vi "SweepOver.vi"(0 "VISA resource name":refnum<visa-resource-name>="LIA", 1 "Sweep Over":string(combo)="Internal Freq", 2 "Sweep Mode":string(combo)="Logarithmic", 3 "End Mode":string(combo)="0", 5 "error in (no error)":errorcluster, 6 "SubVI":bool, 7 "Sweep Time":dbl=100.0 min=0.0 format="%#.4g", 8 "?":bool, 9 "Update Interval":string(combo)="0", 10 "Single Lock-in Parameter 1 (0: X output)":i32(ring)=15 items=["X output", "Y output", "R output", "Theta output", "Aux In 1", "Aux In 2", "Aux In 3", "Aux In 4", "Aux Out 1", "Aux Out 2", "Xnoise", "Ynoise", "Reference Phase", "Sine Out Amplitude", "DC Level", "Int. Ref. Frequency", "Ext. Ref. Frequency"], 11 "Sweep Start":dbl=0.001 min=0.001 max=2500000.0, 12 "Single Lock-in Parameter 2 (0: X output)":i32(ring)=2 items=["X output", "Y output", "R output", "Theta output", "Aux In 1", "Aux In 2", "Aux In 3", "Aux In 4", "Aux Out 1", "Aux Out 2", "Xnoise", "Ynoise", "Reference Phase", "Sine Out Amplitude", "DC Level", "Int. Ref. Frequency", "Ext. Ref. Frequency"], 13 "Sweep End":dbl=2500000.0 min=0.001 max=2500000.0) -> (14 "VISA resource name out":refnum<visa-resource-name>, 15 "output cluster":cluster{dbl[], dbl[]}, 19 "error out":errorcluster)   [LabVIEW 2016]
uses:
  <instrlib>/Stanford Research SR865/Stanford Research SR865.lvlib
panel:
  out "Scan State 2":i32(ring) items=["Off or Disabled", "Reset", "Running", "Paused", "Done"]
  out "?":string="Hz"
  out "?":string="Hz"
  # "s"
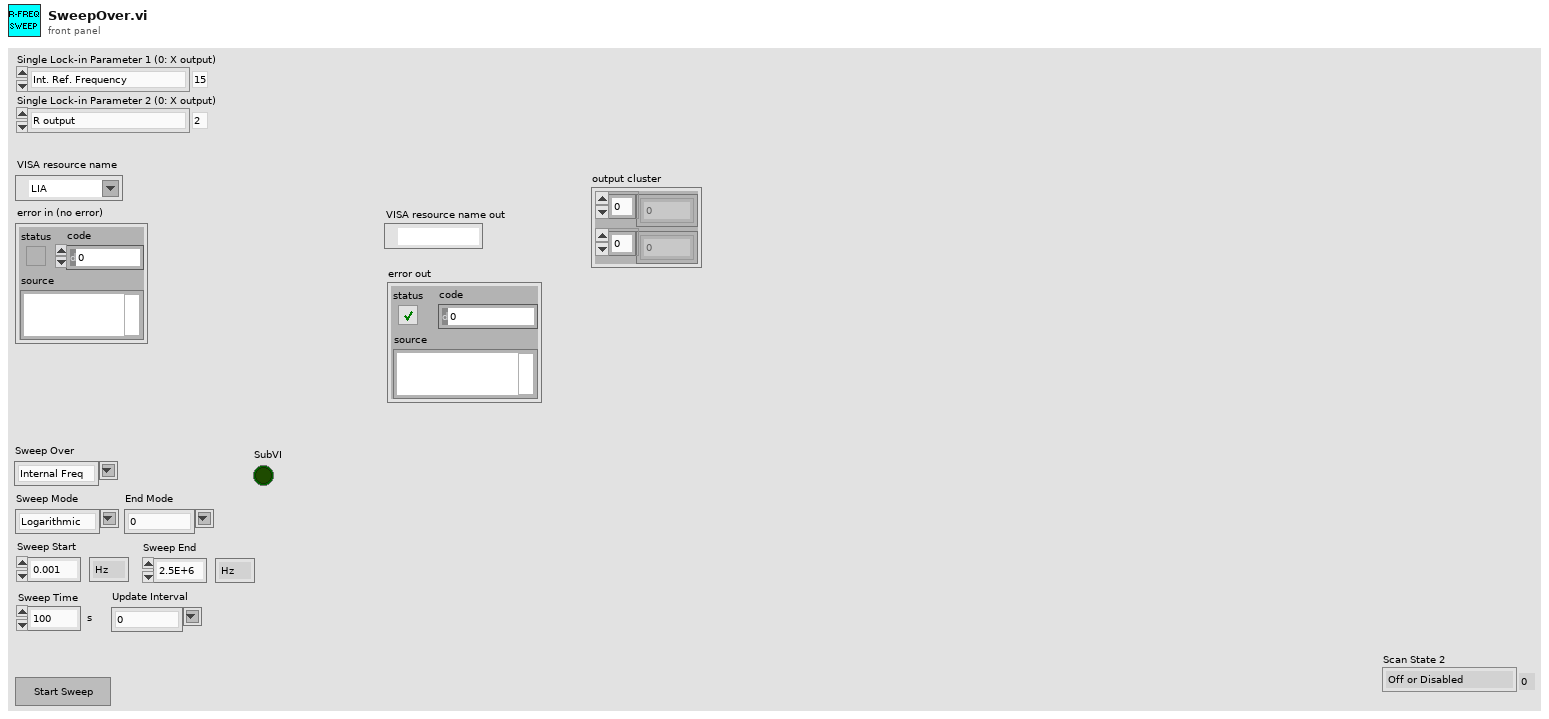
[diagram p1: front panel]
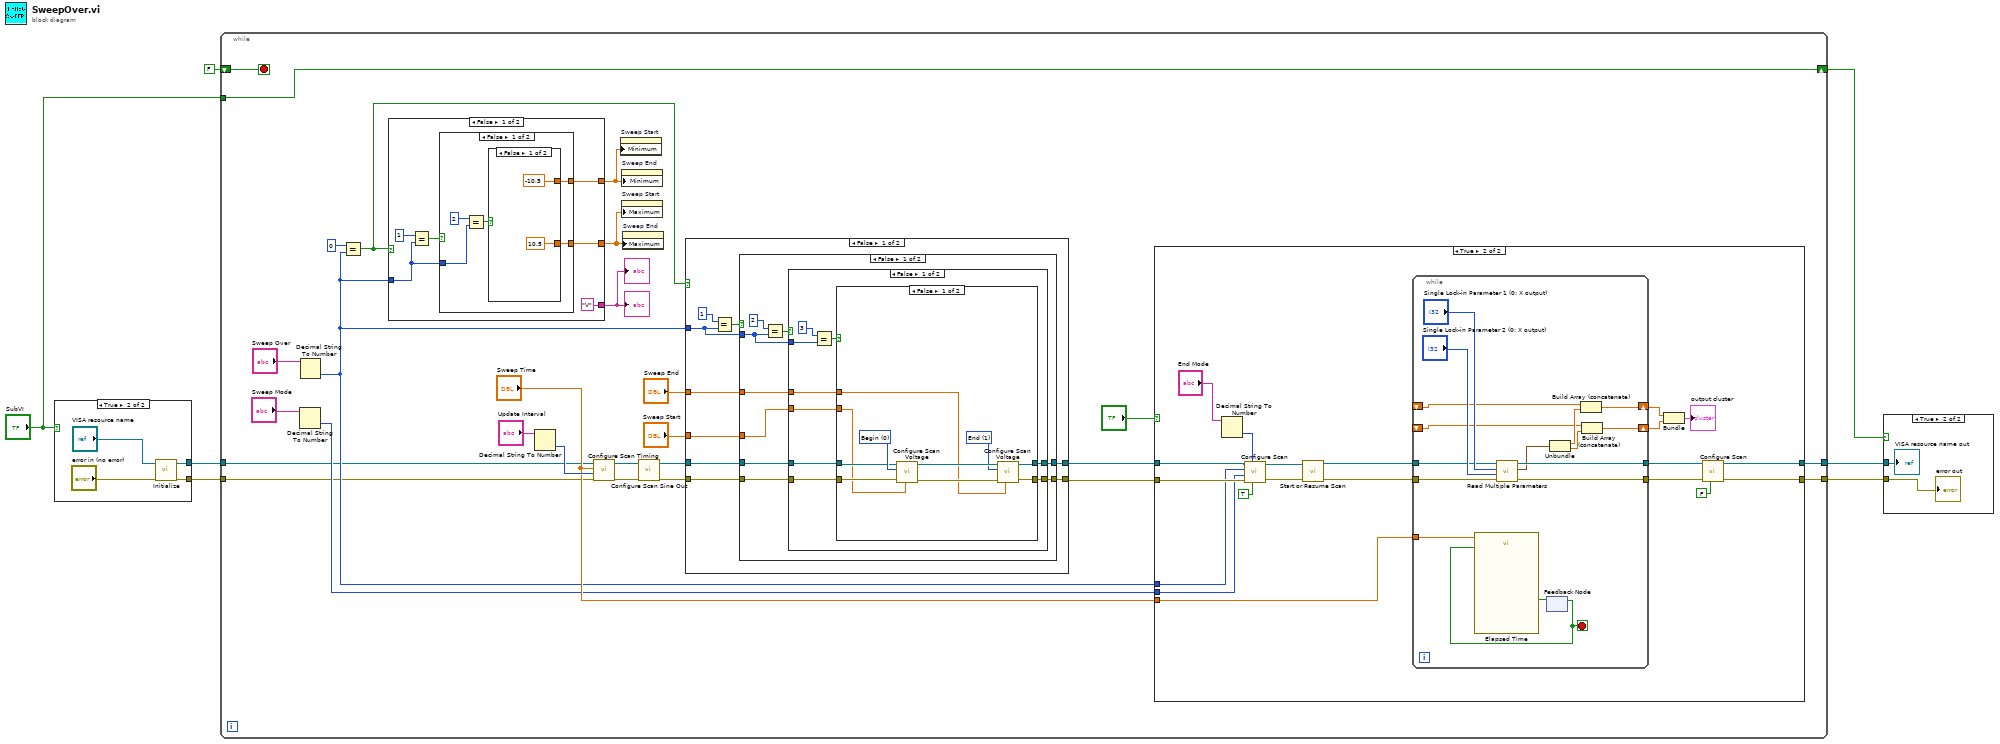
[diagram p0: block diagram]
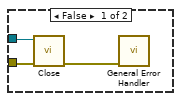
[diagram p2: hidden frame]
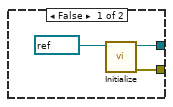
[diagram p3: hidden frame]
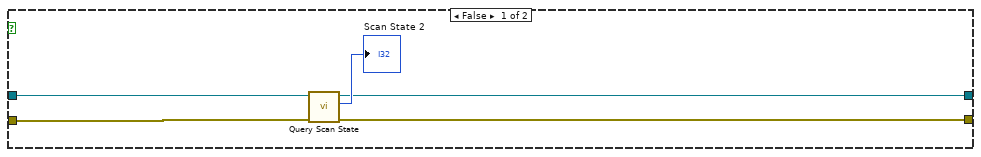
[diagram p4: hidden frame]
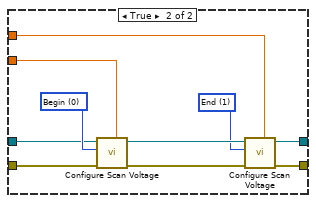
[diagram p5: hidden frame]
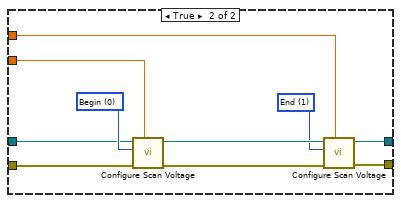
[diagram p6: hidden frame]
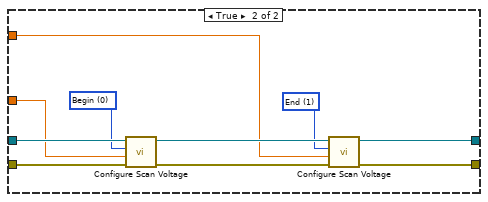
[diagram p7: hidden frame]
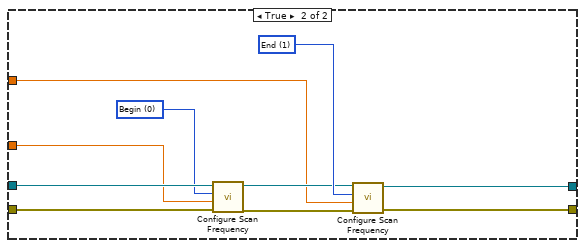
[diagram p8: hidden frame]
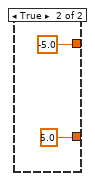
[diagram p9: hidden frame]
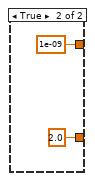
[diagram p10: hidden frame]
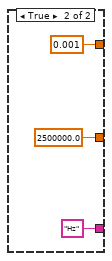
[diagram p11: hidden frame]
diagram:
  n1 = case shown="True" "SubVI" {
    tunnel: [w9 w14] -> w7
    tunnel: [w8 w13] -> w6
    frame False {
      n2 = call <instrlib>:"Initialize.vi"("VISA resource name"=refnum<visa-resource-name> "LIA") -> ("error out"=w8:errorcluster, "VISA resource name out"=w9:refnum<visa-resource-name>)  [unwired: 9 in]
    }
    frame True {
      n3 = call <instrlib>:"Initialize.vi"("error in (no error)"="error in (no error)", "VISA resource name"="VISA resource name") -> ("error out"=w13:errorcluster, "VISA resource name out"=w14:refnum<visa-resource-name>)  [unwired: 8 in]
    }
  }
  n4 = while {
    tunnel: w7 -> [w18]
    tunnel: w6 -> [w17]
    tunnel: [w25] -> w3
    tunnel: [w24] -> w4
    shift-right: [w15] -> w1
    shift-left: FALSE ("SubVI") -> [w23]
    tunnel: "SubVI" -> [w15]
    stop <- w23 stop-if-true
    n5 = Decimal String To Number(string="Sweep Mode") -> (number=w19:i32)  [unwired: 2 in, 1 out]
    n6 = Decimal String To Number(string="Sweep Over") -> (number=w20:i32)  [unwired: 2 in, 1 out]
    n7 = Equal?(x=0, y=w20) -> (x = y?=w29:bool)
    n8 = case shown="False" w29 {
      tunnel: ["V" "Hz"] -> w32
      tunnel: w20 -> [w160 _]
      tunnel: [w162 0.001 ("Data Entry Limits:Minimum")] -> w28
      tunnel: [w161 2500000.0 ("Data Entry Limits:Maximum")] -> w27
      frame False {
        n9 = Equal?(x=1, y=w160) -> (x = y?=w163:bool)
        n10 = case shown="False" w163 {
          tunnel: [w170 1e-09 ("Data Entry Limits:Maximum")] -> w162
          tunnel: [w169 2.0 ("Data Entry Limits:Minimum")] -> w161
          tunnel: w160 -> [w167 _]
          frame False {
            n11 = Equal?(x=2, y=w167) -> (x = y?=w166:bool)
            n12 = case shown="False" w166 {
              tunnel: [-10.5 ("Data Entry Limits:Maximum") -5.0 ("Data Entry Limits:Maximum")] -> w170
              tunnel: [10.5 ("Data Entry Limits:Minimum") 5.0 ("Data Entry Limits:Minimum")] -> w169
              frame False {
              }
              frame True {
              }
            }
          }
          frame True {
          }
        }
      }
      frame True {
      }
    }
    "?" <- w32
    "?" <- w32
    n13 = Decimal String To Number(string="Update Interval") -> (number=w35:i32)  [unwired: 2 in, 1 out]
    n14 = call <instrlib>:"Configure Scan Timing.vi"("error in (no error)"=w17, "Update Interval (0: 8ms)"=w35, "Scan Time (100)"="Sweep Time", "VISA resource name"=w18) -> ("error out"=w40:errorcluster, "VISA resource name out"=w41:refnum<visa-resource-name>)  [unwired: 6 in]
    n15 = property on="Sweep Start" class="DigNum (strict)"("Minimum"=w28) -> ()  [unwired: 2 in, 2 out]
    n16 = property on="Sweep End" class="DigNum (strict)"("Minimum"=w28) -> ()  [unwired: 2 in, 2 out]
    n17 = property on="Sweep Start" class="DigNum (strict)"("Maximum"=w27) -> ()  [unwired: 2 in, 2 out]
    n18 = property on="Sweep End" class="DigNum (strict)"("Maximum"=w27) -> ()  [unwired: 2 in, 2 out]
    n19 = call <instrlib>:"Configure Scan Sine Out.vi"("error in (no error)"=w40, "VISA resource name"=w41) -> ("error out"=w38:errorcluster, "VISA resource name out"=w39:refnum<visa-resource-name>)  [unwired: 8 in]
    n20 = case shown="False" w29 {
      tunnel: w39 -> [w91 w159]
      tunnel: w38 -> [w90 w158]
      tunnel: [w89 w153] -> w22
      tunnel: [w88 w152] -> w21
      tunnel: "Sweep Start" -> [w84 w151]
      tunnel: "Sweep End" -> [w85 w150]
      tunnel: w20 -> [w83 _]
      frame False {
        n21 = Equal?(x=1, y=w83) -> (x = y?=w86:bool)
        n22 = case shown="False" w86 {
          tunnel: w91 -> [w100 w149]
          tunnel: w90 -> [w99 w148]
          tunnel: [w98 w145] -> w89
          tunnel: [w97 w144] -> w88
          tunnel: w85 -> [w93 w140]
          tunnel: w84 -> [w94 w141]
          tunnel: w83 -> [w92 _]
          frame False {
            n23 = Equal?(x=2, y=w92) -> (x = y?=w95:bool)
            n24 = case shown="False" w95 {
              tunnel: w100 -> [w103 w135]
              tunnel: w99 -> [w104 w134]
              tunnel: [w106 w133] -> w98
              tunnel: [w105 w132] -> w97
              tunnel: w94 -> [w102 w131]
              tunnel: w93 -> [w101 w130]
              tunnel: w92 -> [w108 _]
              frame False {
                n25 = Equal?(x=3, y=w108) -> (x = y?=w107:bool)
                n26 = case shown="False" w107 {
                  tunnel: [w114 w125] -> w106
                  tunnel: [w115 w124] -> w105
                  tunnel: w104 -> [w112 w123]
                  tunnel: w103 -> [w113 w122]
                  tunnel: w102 -> [w111 w121]
                  tunnel: w101 -> [w110 w120]
                  frame False {
                    w116 = 1 items=["Begin", "End"] ("Scan Begin or End (0: Begin)")
                    w117 = 0 items=["Begin", "End"] ("Scan Begin or End (0: Begin)")
                    n27 = call <instrlib>:"Configure Scan Voltage.vi"("AuxOut2 to Voltage (2)"=w111, "error in (no error)"=w112, "Scan Begin or End (0: Begin)"=w117, "VISA resource name"=w113) -> ("error out"=w119:errorcluster, "VISA resource name out"=w118:refnum<visa-resource-name>)  [unwired: 6 in]
                    n28 = call <instrlib>:"Configure Scan Voltage.vi"("AuxOut2 to Voltage (2)"=w110, "error in (no error)"=w119, "Scan Begin or End (0: Begin)"=w116, "VISA resource name"=w118) -> ("error out"=w115:errorcluster, "VISA resource name out"=w114:refnum<visa-resource-name>)  [unwired: 6 in]
                  }
                  frame True {
                    w126 = 1 items=["Begin", "End"] ("Scan Begin or End (0: Begin)")
                    w127 = 0 items=["Begin", "End"] ("Scan Begin or End (0: Begin)")
                    n29 = call <instrlib>:"Configure Scan Voltage.vi"("AuxOut 1 to Voltage (-2)"=w121, "error in (no error)"=w123, "Scan Begin or End (0: Begin)"=w127, "VISA resource name"=w122) -> ("error out"=w129:errorcluster, "VISA resource name out"=w128:refnum<visa-resource-name>)  [unwired: 6 in]
                    n30 = call <instrlib>:"Configure Scan Voltage.vi"("AuxOut 1 to Voltage (-2)"=w120, "error in (no error)"=w129, "Scan Begin or End (0: Begin)"=w126, "VISA resource name"=w128) -> ("error out"=w124:errorcluster, "VISA resource name out"=w125:refnum<visa-resource-name>)  [unwired: 6 in]
                  }
                }
              }
              frame True {
                w136 = 1 items=["Begin", "End"] ("Scan Begin or End (0: Begin)")
                w137 = 0 items=["Begin", "End"] ("Scan Begin or End (0: Begin)")
                n31 = call <instrlib>:"Configure Scan Voltage.vi"("DC Level to Voltage (-1)"=w131, "error in (no error)"=w134, "Scan Begin or End (0: Begin)"=w137, "VISA resource name"=w135) -> ("error out"=w139:errorcluster, "VISA resource name out"=w138:refnum<visa-resource-name>)  [unwired: 6 in]
                n32 = call <instrlib>:"Configure Scan Voltage.vi"("DC Level to Voltage (-1)"=w130, "error in (no error)"=w139, "Scan Begin or End (0: Begin)"=w136, "VISA resource name"=w138) -> ("error out"=w132:errorcluster, "VISA resource name out"=w133:refnum<visa-resource-name>)  [unwired: 6 in]
              }
            }
          }
          frame True {
            w142 = 1 items=["Begin", "End"] ("Scan Begin or End (0: Begin)")
            w143 = 0 items=["Begin", "End"] ("Scan Begin or End (0: Begin)")
            n33 = call <instrlib>:"Configure Scan Voltage.vi"("error in (no error)"=w148, "Amplitude to Voltage (1)"=w141, "Scan Begin or End (0: Begin)"=w143, "VISA resource name"=w149) -> ("error out"=w147:errorcluster, "VISA resource name out"=w146:refnum<visa-resource-name>)  [unwired: 6 in]
            n34 = call <instrlib>:"Configure Scan Voltage.vi"("error in (no error)"=w147, "Amplitude to Voltage (1)"=w140, "Scan Begin or End (0: Begin)"=w142, "VISA resource name"=w146) -> ("error out"=w144:errorcluster, "VISA resource name out"=w145:refnum<visa-resource-name>)  [unwired: 6 in]
          }
        }
      }
      frame True {
        w156 = 1 items=["Begin", "End"] ("Scan Begin or End (0: Begin)")
        w157 = 0 items=["Begin", "End"] ("Scan Begin or End (0: Begin)")
        n35 = call <instrlib>:"Configure Scan Frequency.vi"("error in (no error)"=w158, "Frequency (100000)"=w151, "Scan Begin or End (0: Begin)"=w157, "VISA resource name"=w159) -> ("error out"=w154:errorcluster, "VISA resource name out"=w155:refnum<visa-resource-name>)  [unwired: 6 in]
        n36 = call <instrlib>:"Configure Scan Frequency.vi"("error in (no error)"=w154, "Frequency (100000)"=w150, "Scan Begin or End (0: Begin)"=w156, "VISA resource name"=w155) -> ("error out"=w152:errorcluster, "VISA resource name out"=w153:refnum<visa-resource-name>)  [unwired: 6 in]
      }
    }
    n37 = case shown="True" "?" {
      tunnel: "Sweep Time" -> [_ w65]
      tunnel: [w42 w52] -> w25
      tunnel: [w43 w51] -> w24
      tunnel: w22 -> [w45 w62]
      tunnel: w21 -> [w44 w61]
      tunnel: w20 -> [_ w60]
      tunnel: w19 -> [_ w59]
      frame False {
        n38 = call <instrlib>:"Query Scan State.vi"("error in (no error)"=w44, "VISA resource name"=w45) -> ("error out"=w43:errorcluster, "Scan State"=→"Scan State 2":i32, "VISA resource name out"=w42:refnum<visa-resource-name>)  [unwired: 7 in]
      }
      frame True {
        n39 = Decimal String To Number(string="End Mode") -> (number=w58:i32)  [unwired: 2 in, 1 out]
        n40 = call <instrlib>:"Configure Scan.vi"("Scanning State (0: Off)"=TRUE, "Scan End Mode (0: Once)"=w58, "error in (no error)"=w61, "Scan Type (0: Linear)"=w59, "Scan Parameter (0: Fint)"=w60, "VISA resource name"=w62) -> ("error out"=w64:errorcluster, "VISA resource name out"=w63:refnum<visa-resource-name>)  [unwired: 4 in]
        n41 = call <instrlib>:"Start or Resume Scan.vi"("error in (no error)"=w64, "VISA resource name"=w63) -> ("error out"=w47:errorcluster, "VISA resource name out"=w48:refnum<visa-resource-name>)  [unwired: 8 in]
        n42 = while {
          tunnel: w65 -> [w80]
          tunnel: [w78] -> w50
          tunnel: [w79] -> w49
          shift-right: [w72] -> w56
          shift-left: _ -> [w69]
          shift-right: [w71] -> w55
          shift-left: _ -> [w70]
          tunnel: w48 -> [w68]
          tunnel: w47 -> [w67]
          stop <- w81 stop-if-true
          n43 = call <instrlib>:"Read Multiple Parameters.vi"("error in (no error)"=w67, "Single Lock-in Parameter 2 (0: X output)"="Single Lock-in Parameter 2 (0: X output)", "Single Lock-in Parameter 1 (0: X output)"="Single Lock-in Parameter 1 (0: X output)", "VISA resource name"=w68) -> ("error out"=w79:errorcluster, "Output Value(2 parameters)"=w75:cluster{"Value 1":dbl, "Value 2":dbl}, "VISA resource name out"=w78:refnum<visa-resource-name>)  [unwired: 4 in, 1 out]
          n44 = feedback #1() -> (w81:bool)  [unwired: 1 in]
          n45 = call "Elapsed Time"("Time Target (s)"=w80, "Reset"=w81) -> ("Time has Elapsed"=w82:bool)  [unwired: 10 in, 7 out]
          n46 = feedback-in #1(w82) -> ()
          n47 = Unbundle(w75) -> ("Value 1"=w74:dbl, "Value 2"=w73:dbl)
          n48 = Build Array (concatenate)(w70, w74) -> (w71:dbl[])
          n49 = Build Array (concatenate)(w69, w73) -> (w72:dbl[])
        }
        n50 = Bundle(w55, w56) -> (→"output cluster":cluster{dbl[], dbl[]})  [unwired: 1 in]
        n51 = call <instrlib>:"Configure Scan.vi"("Scanning State (0: Off)"=FALSE, "error in (no error)"=w49, "VISA resource name"=w50) -> ("error out"=w51:errorcluster, "VISA resource name out"=w52:refnum<visa-resource-name>)  [unwired: 7 in]
      }
    }
  }
  n52 = case shown="True" w1 {
    tunnel: w4 -> [w180 w183]
    tunnel: w3 -> [w181 w184]
    frame False {
      n53 = call <instrlib>:"Close.vi"("error in (no error)"=w180, "VISA resource name"=w181) -> ("error out"=w182:errorcluster)  [unwired: 9 in]
      n54 = call <vilib>:"General Error Handler.vi"("error in (no error)"=w182) -> ()  [unwired: 10 in, 5 out]
    }
    frame True {
      "VISA resource name out" <- w184
      "error out" <- w183
    }
  }
